vi "S2C_FORNAX_Poly_DftAlarmCommand.vi"(8 "Error In":errorcluster, 10 "DftAlarmCommand":T5={"Partition"="Default", "Message"="DftAlarmCommand", "M_ModuleId"=0, "M_AlarmCode"=0, "M_Command"=0, "M_EnergyChannelId"=0, "M_Message"="", "M_CommandParams"="", "M_CommandOptions"=""} {"M_EnergyChannelId" items=["EC_MONO_1"=0, "EC_BIPOLAR"=1, "EC_MONO_2"=2, "EC_ADVANCED"=3, "EC_ADVANCED_ECUT"=4, "EC_ADVANCED_DCUT"=5, "EC_SHARED_COAG"=6, "EC_INTERNAL_BIP_CAL"=7, "EC_NOT_USED"=-1]; "M_Command" items=["DFT_ALARM_COMMAND_INVALID", "DFT_ALARM_RAISE_START", "DFT_ALARM_RAISE_STOP", "DFT_ALARM_RAISE_ONCE", "NUM_DFT_ALARM_COMMANDS"]; "M_AlarmCode" items=["INFO_LOGGING"=0, "BPC_FPGA_FAILURE"=101, "PERC_FPGA_FAILURE"=102, "RIGEL_FPGA_FAILURE"=103, "BOOT_SECTOR_FAILURE"=104, "RAM_TEST_FAILURE"=105, "PROCESSOR_EXCEPTION"=106, "UNKNOWN_INTERRUPT"=107, "SSD_FLASH_FAILURE"=201, "RTOS_FAILURE"=202, "OS_FAILURE"=203, "ASSERT"=204, "NULL_POINTER"=205, "DATABASE_ERROR"=206, "MEM_ALLOCATE_ERROR"=207, "STACK_OVERFLOW"=208, "DMA_FAILURE"=209, "MAX_THREAD_LIMIT"=210, "DDS_FAILURE"=211, "CONTROLLER_PCBA_FAILURE"=212, "SR_PCBA_FAILURE"=213, "RF_PCBA_FAILURE"=214, "INVALID_SOFTWARE_STATE"=215, "LVDC_RAIL_FAILURE"=216, "HVDC_RAIL_FAILURE"=217, "DISPLAY_DRIVER_ERROR"=218, "AUDIO_CIRCUIT_FAILURE"=219, "MULTI_TASKING_ERROR"=220, "CAMM_TIMEBASE_ERROR"=221, "EM_TIMEBASE_ERROR"=222, "BPC_TIMEBASE_ERROR"=223, "PERC_TIMEBASE_ERROR"=224, "CAMM_WATCHDOG_ERROR"=225, "BPC_COMM_FAILURE"=226, "REM_CIRCUIT_FAILURE"=227, "RELAY_FEEDBACK_FAILURE"=228, "CONNECTOR_DIAGNOSTIC_FAILURE"=229, "CRITICAL_DATA_FAILURE"=230, "SECURITY_ACCESS_ERROR"=231, "INVALID_SYSTEM_CONFIGURATION"=232, "FRU_UPDATED_REDOCK"=233, "EM_COMM_FAILURE"=234, "REM_FAILURE"=235, "CLP_WATCHDOG_ERROR"=236, "SOFTWARE_FAILURE"=238, "INVALID_VALUE"=239, "THREAD_CHECK_FAILURE"=240, "HIGH_RF_DATA_CORRUPTION_RATE"=241, "RF_DATA_TIMING_VARIANCE"=242, "RF_DATA_DELAY"=243, "RF_INTERRUPT_VARIANCE"=244, "HWC_CONTROL_SELECTION"=246, "HVPS_PCBA_FAILURE"=247, "FP_PCBA_FAILURE"=248, "RTC_FAILURE"=249, "RJ45_DIAGNOSTIC_FAIL"=301, "MONO_1_IF_COMM_FAIL"=302, "MONO_2_IF_COMM_FAIL"=303, "BIP_IF_COMM_FAIL"=304, "LIG_IF_COMM_FAIL"=305, "LIG_VIBE_FAIL"=306, "UNSUPPORTED_COMMAND"=307, "SOFTWARE_TIMEOUT"=308, "ACTIVATION_DENIED"=309, "TOUCHSCREEN_STUCK"=310, "ABSOLUTE_INTEGRATED_ERROR"=312, "VOLTAGE_SENSOR_COMPARE_ERROR"=313, "CURRENT_SENSOR_COMPARE_ERROR"=314, "SENSOR_POWER_COMPARE_ERROR"=315, "IEC_POWER_COMPARE_ERROR"=316, "MAXIMUM_PVI_CONTROL_CURVE_COMPARE_ERROR"=317, "VOLTAGE_SENSOR_CLIP_ERROR"=318, "CURRENT_SENSOR_CLIP_ERROR"=319, "MONO_1_HANDSWITCH_STUCK"=320, "MONO_1_FOOTSWITCH_STUCK"=321, "MONO_2_HANDSWITCH_STUCK"=322, "MONO_2_FOOTSWITCH_STUCK"=323, "BIP_HANDSWITCH_STUCK"=324, "BIP_FOOTSWITCH_STUCK"=325, "LIG_HANDSWITCH_STUCK"=326, "LIG_FOOTSWITCH_STUCK"=327, "FP_BUTTON_STUCK"=328, "INVALID_FOOTSWITCH_INPUT"=329, "PROLONGED_ACTIVATION"=330, "INVALID_INSTRUMENT"=331, "CHASSIS_OVERTEMP"=332, "FAN_FAILURE"=333, "REM_CHECK_FAILURE"=334, "PROC_FILE_OPEN_FAILURE"=335, "ADC_SYNC_ERROR"=336, "REAL_TIME_CLOCK_FAIL"=337, "LIMIT_CHECK_FAILURE"=339, "INSTALL_COUNTRY_CODE"=340, "UI_SPI_COMM_FAIL"=341, "FS_SPI_COMM_FAIL"=342, "REM_SPI_RX_ERROR"=343, "REM_SPI_TX_ERROR"=344, "REM_I2C_RX_ERROR"=345, "REM_I2C_TX_ERROR"=346, "REM_DATA_ERROR"=347, "ASSERT_NON_CRITICAL"=348, "THREAD_CHECK_FAILURE_NON_CRITICAL"=349, "RETURN_ELECTRODE_OVERTEMP"=350, "ISOFIRM_WATCHDOG_ERROR"=351, "SW_FPGA_UPDATE_FAIL"=352, "TS_CAL_RESET"=353, "SWC_TARGET_VARIANCE"=354, "FOOTPEDAL_NOT_SUPPORTED"=355, "INVALID_RF_CALIBRATION"=356, "USE_RESTRICTION_COMM_ERROR"=357, "SECURITY_ACCESS_NOTIFICATION"=401, "SEAL_CYCLE_INTERRUPTED"=402, "SEAL_SHORT_CIRCUIT"=403, "SEAL_OPEN_CIRCUIT"=404, "SEAL_TIMEOUT"=405, "MONO_2_BOTH_PLUGS"=407, "LIG_BOTH_PLUGS"=408, "INVALID_ACTIVATE_MONO_2_BOTH_PLUGS"=411, "INVALID_ACTIVATE_LIG_BOTH_PLUGS"=412, "MONO_2_COMBINATION_NOT_ALLOWED"=413, "LIG_COMBINATION_NOT_ALLOWED"=414, "FEATURE_NOT_ENABLED"=415, "INSTRUMENT_NOT_DETECTED"=416, "INSTRUMENT_NOT_COMPATIBLE"=417, "STARTING_ABP_Z_TOO_LOW"=419, "INSTRUMENT_USAGE_LIMIT_CANNOT_CONTINUE"=420, "INSTRUMENT_USAGE_LIMIT_CAN_CONTINUE"=421, "BIPOLAR_CABLE_NOT_DETECTED"=422, "AUTOBIPOLAR_TURNED_OFF"=423, "AUTOBIPOLAR_CYCLE_TIMEOUT"=424, "WAITING_FOR_ABP_OPEN_CIRCUIT"=425, "BIPOLAR_CABLE_NOT_INSERTED"=426, "ABLATION_STOPPED_HIGH_Z"=427, "ABLATION_STOPPED_LOW_Z"=428, "PROLONGED_CARDIO_ABLATION"=429, "PROLONGED_BPR_ACTIVATION"=430, "BPR_STOPPED_HIGH_Z"=431, "SEAL_THICK_TISSUE_INCOMPLETE"=432, "INSTRUMENT_SHELF_LIFE_EXCEEDED"=433, "UNAUTHENTIC_INSTRUMENT"=434, "INSERTION_DETECTION_SWITCH_STUCK"=435, "UNAUTHENTIC_INSTRUMENT_MISMATCH"=436, "USAGE_MISMATCH"=437, "MODEL_PORT_DISABLED"=438, "UNSUPPORTED_INSTRUMENT"=439, "MAX_ALARM_CODE"=500]; "M_ModuleId" items=["MODULE_INVALID"=0, "MODULE_LOG_WRITER"=1, "MODULE_ACTIVATION_MGR"=2, "MODULE_ALARM_MGR"=3, "MODULE_AUDIO_MGR"=4, "MODULE_BPC_INTERFACE"=5, "MODULE_EM_INTERFACE"=6, "MODULE_CLINICAL_GUI_MGR"=7, "MODULE_SERVICE_GUI_MGR"=8, "MODULE_SERVICE_MGR"=9, "MODULE_CONFIGURATION_MGR"=10, "MODULE_EXTERNAL_COMM_MGR"=11, "MODULE_PERSISTENT_DATA_MGR"=12, "MODULE_RF_DATA_WRITER"=13, "MODULE_TEMPERATURE_MGR"=14, "MODULE_TSMONITOR"=15, "MODULE_SUPERVISOR"=16, "MODULE_SW_UPDATE_MGR"=17, "MODULE_EM_BOOT"=18, "MODULE_PERC_PS_HV_CONTROL"=19, "MODULE_END_OF_INTERNAL"=20, "MODULE_EXT_VLEX"=50, "MODULE_EXT_FORNAX"=51, "MODULE_EXT_FW_UPDATE_CLI"=52, "MODULE_EXT_SIMULATOR"=53, "MODULE_BOARD_ID_UTIL"=54, "MODULE_ISO_UTIL"=55, "MODULE_CONFIG_DATA_UTIL"=56, "MODULE_SIM_BPC"=57, "MODULE_SIM_VIBE"=58, "MODULE_CAMM_GUARD"=59, "MODULE_CUSTODIAN"=60, "MODULE_OS_SERVICES_MGR"=61, "NUM_MODULE_IDS"=62]}, 11 "Settings":T6={"Driver"="Fornax", "Command"="DftAlarmCommand", "Return"="ErrorStatus", "Parameters"="", "Timeout"=10.0}) -> (0 "Error Out":errorcluster, 3 "Response":string)   [LabVIEW 2015]
uses:
  Typedefs/ModuleId.ctl
  Typedefs/PhoenixErrors.ctl
  Typedefs/DftAlarmCommand.ctl
  Typedefs/EnergyChannelId.ctl
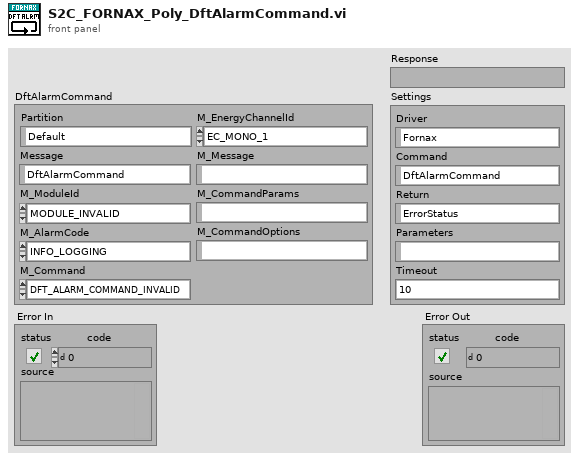
[diagram p1: front panel]
types:
  T1 = typedef "ModuleId.ctl" = i16
  T2 = typedef "PhoenixErrors.ctl" = i16
  T3 = typedef "DftAlarmCommand.ctl" = i16
  T4 = typedef "EnergyChannelId.ctl" = i16
  T5 = cluster{"Partition":string, "Message":string, "M_ModuleId":T1, "M_AlarmCode":T2, "M_Command":T3, "M_EnergyChannelId":T4, "M_Message":string, "M_CommandParams":string, "M_CommandOptions":string}
  T6 = cluster{"Driver":string, "Command":string, "Return":string, "Parameters":string, "Timeout":dbl}
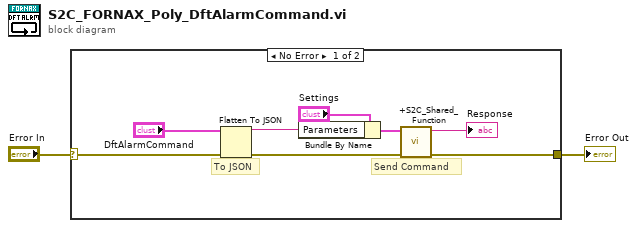
[diagram p0: block diagram]
diagram:
  n1 = case shown="No Error" "Error In" {
    selector: "Error In" -> [w6 w11]
    tunnel: [w5 w11] -> w1
    frame No Error {
      # "To JSON"
      # "Send Command"
      n2 = Flatten To JSON(anything="DftAlarmCommand", error in (no error)=w6) -> (JSON string=w7:string, 11:w9:errorcluster)  [unwired: 1 in]
      n3 = Bundle By Name(cluster="Settings", "Parameters"=w7) -> (w10:T6)
      n4 = call "+S2C_Shared_Function.vi"("Error In"=w9, "Settings"=w10) -> ("Error Out"=w5:errorcluster, "Response"=→"Response":string)  [unwired: 8 in]
    }
    frame Error {
    }
  }
  "Error Out" <- w1
